vi "FFTs.vi"(8 "error in":errorcluster, 9 "Envelope&Hu?":bool, 10 "duration":dbl=20.0 format="%#_13g", 11 "waveform in":waveform(dbl)) -> (0 "error out":errorcluster, 3 "output cluster":T1)   [LabVIEW 2025]
uses:
  <vilib>/Analysis/2dsp.llb/Real FFT.vi
  <vilib>/Waveform/WDTOps.llb/WDT Waveform Duration DBL.vi
  <vilib>/Waveform/WDTOps.llb/WDT Get Waveform Subset DBL.vi
  <vilib>/Analysis/NI_AALPro.lvlib
panel:
  out "freq_array":dbl[](array[numeric])
  out "Huell_spec":dbl[](array[numeric])
  out "freq_step":dbl
  out "Envelope":dbl[](array[numeric])
  out "abs_FFT":dbl[](array[numeric])
  out "Rohdaten":waveform(dbl)
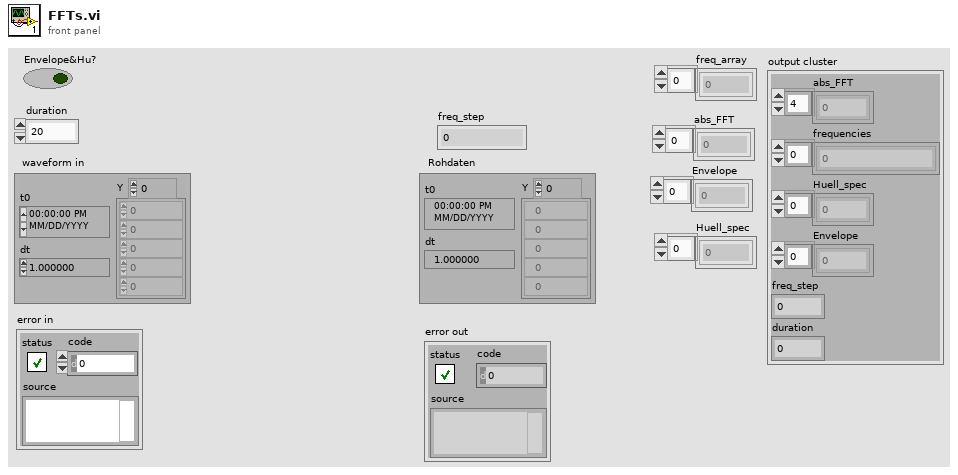
[diagram p1: front panel]
types:
  T1 = cluster{"abs_FFT":dbl[], "frequencies":dbl[], "Huell_spec":dbl[], "Envelope":dbl[], "freq_step":dbl, "duration":dbl}
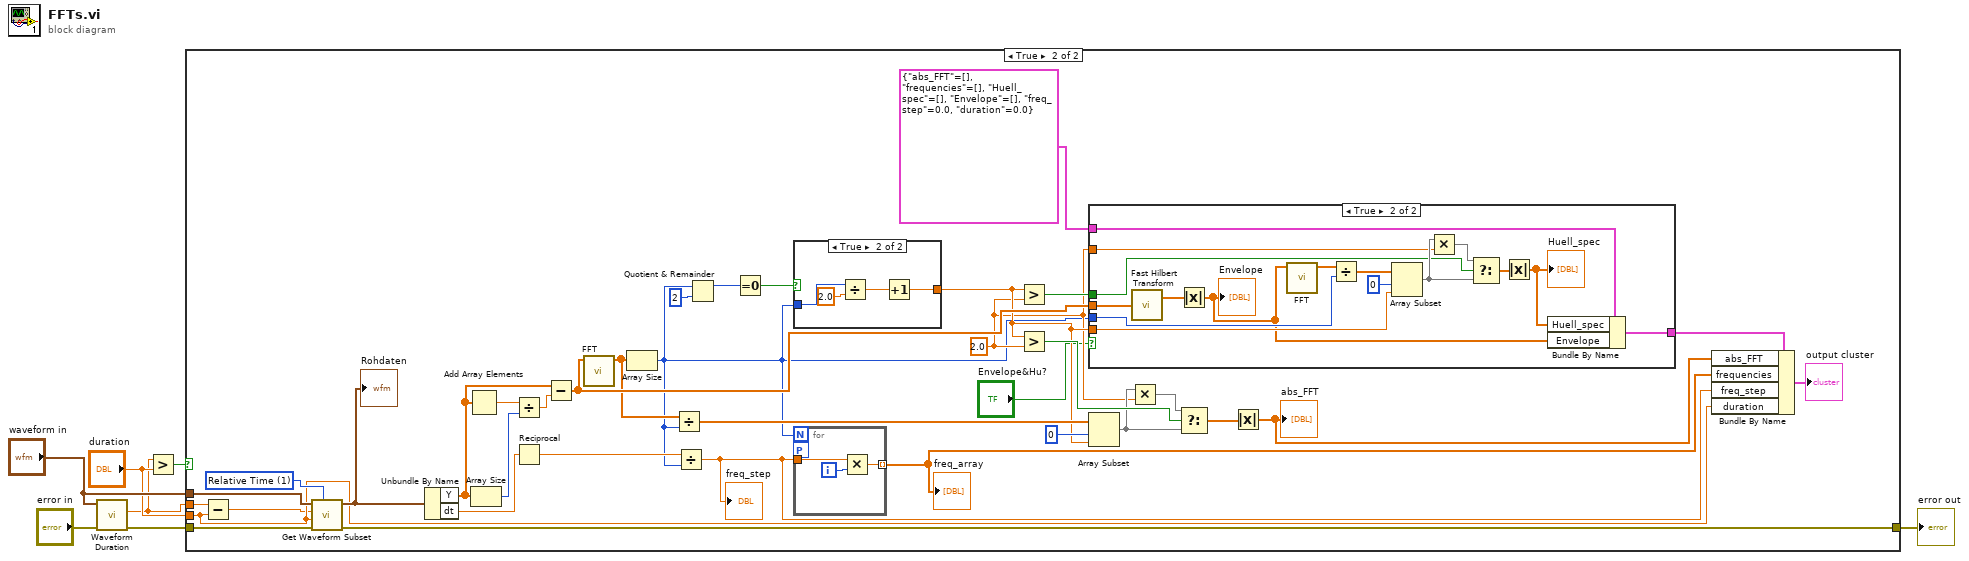
[diagram p0: block diagram]
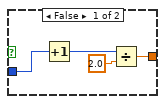
[diagram p4: hidden frame]
diagram:
  n1 = call-poly <vilib>:"Waveform Duration.vi"("error in (no error)"="error in", "waveform in"="waveform in") -> ("error out"=w4:errorcluster, "duration"=w1:dbl)  [unwired: 7 in, 1 out]
  n2 = Greater?(x=w1, y="duration") -> (0:w6:bool)
  n3 = case shown="True" w6 {
    tunnel: "waveform in" -> [_ w14]
    tunnel: "duration" -> [_ w11]
    tunnel: w4 -> [w8 w13]
    tunnel: [w8 w25] -> w3
    tunnel: w1 -> [_ w12]
    frame False {
    }
    frame True {
      w24 = 2.0 ("y")
      w44 = u16 1 items=["Samples", "Relative Time"] ("start/duration format")
      n4 = Subtract(x=w12, y=w11) -> (x-y=w10:dbl)
      n5 = call-poly <vilib>:"Get Waveform Subset.vi"("start/duration format"=w44, "error in (no error)"=w13, "duration"=w11, "start samples/time"=w10, "waveform in"=w14) -> ("error out"=w25:errorcluster, "waveform out"=w38:waveform(dbl))  [unwired: 1 in, 2 out]
      "Rohdaten" <- w38
      n6 = Unbundle By Name(w38) -> ("Y"=w39:dbl[], "dt"=w9:dbl)
      n7 = Add Array Elements(numeric array=w39) -> (sum=w43:dbl)
      n8 = Array Size(array=w39) -> (size(s)=w40:i32)
      n9 = Divide(x=w43, y=w40) -> (x/y=w42:dbl)
      n10 = Reciprocal(x=w9) -> (1/x=w20:dbl)
      n11 = Subtract(x=w39, y=w42) -> (x-y=w41:dbl[])
      n12 = call-poly <vilib>:"FFT.vi"("X"=w41) -> ("FFT {X}"=w32:cdb[])  [unwired: 9 in, 1 out]
      n13 = Array Size(array=w32) -> (size(s)=w19:i32)
      n14 = Divide(x=w32, y=w19) -> (x/y=w31:cdb[])
      n15 = Divide(x=w20, y=w19) -> (x/y=w15:dbl)
      "freq_step" <- w15
      n16 = Quotient & Remainder(x=w19, y=2) -> (x-y*floor(x/y)=w35:i32)  [unwired: 1 out]
      n17 = Equal To 0?(x=w35) -> (x = 0?=w34:bool)
      n18 = case shown="True" w34 {
        tunnel: w19 -> [w67 w70]
        tunnel: [w65 w69] -> w26
        frame False {
          n19 = Increment(x=w67) -> (x+1=w66:i32)
          n20 = Divide(x=w66, y=2.0) -> (x/y=w65:dbl)
        }
        frame True {
          n21 = Divide(x=w70, y=2.0) -> (x/y=w72:dbl)
          n22 = Increment(x=w72) -> (x+1=w69:dbl)
        }
      }
      n23 = for {
        N: w19 -> [_]
        tunnel: w15 -> [w64]
        tunnel: [w62] -> w23 mode=indexing
        workers-P: _ -> [_]
        i -> [w63]
        n24 = Multiply(x=w64, y=w63) -> (x*y=w62:dbl)
      }
      "freq_array" <- w23
      n25 = Greater?(x=w26, y=w24) -> (0:w27:bool)
      n26 = Greater?(x=w26, y=w24) -> (0:w33:bool)
      n27 = case shown="True" "Envelope&Hu?" {
        tunnel: w41 -> [_ w61]
        tunnel: w27 -> [_ w56]
        tunnel: w26 -> [_ w52]
        tunnel: w24 -> [_ w51]
        tunnel: w19 -> [_ w50]
        tunnel: T1 {"abs_FFT"=[], "frequencies"=[], "Huell_spec"=[], "Envelope"=[], "freq_step"=0.0, "duration"=0.0} -> [w45 w49]
        tunnel: [w45 w46] -> w17
        frame False {
        }
        frame True {
          n28 = call <vilib>:"Fast Hilbert Transform.vi"("X"=w61) -> ("Hilbert{X}"=w60:dbl[])  [unwired: 1 out]
          n29 = Absolute Value(x=w60) -> (abs(x)=w47:dbl[])
          "Envelope" <- w47
          n30 = call-poly <vilib>:"FFT.vi"("X"=w47) -> ("FFT {X}"=w53:cdb[])  [unwired: 9 in, 1 out]
          n31 = Divide(x=w53, y=w50) -> (x/y=w54:cdb[])
          n32 = Array Subset(array=w54, index=0, length=w52) -> (w58:cdb[])
          n33 = Multiply(x=w58, y=w51) -> (x*y=w57:cdb[])
          n34 = Select(t=w57, s=w56, f=w58) -> (s? t:f=w59:cdb[])
          n35 = Absolute Value(x=w59) -> (abs(x)=w48:dbl[])
          "Huell_spec" <- w48
          n36 = Bundle By Name(cluster=w49, "Huell_spec"=w48, "Envelope"=w47) -> (w46:T1)
        }
      }
      n37 = Array Subset(array=w31, index=0, length=w26) -> (w29:cdb[])
      n38 = Multiply(x=w29, y=w24) -> (x*y=w30:cdb[])
      n39 = Select(t=w30, s=w33, f=w29) -> (s? t:f=w28:cdb[])
      n40 = Absolute Value(x=w28) -> (abs(x)=w22:dbl[])
      "abs_FFT" <- w22
      n41 = Bundle By Name(cluster=w17, "abs_FFT"=w22, "frequencies"=w23, "freq_step"=w15, "duration"=w11) -> (→"output cluster":T1)
    }
  }
  "error out" <- w3
